vi "5492_WPI_RobotDriveArcadeDrive_Standard(NoSaturation).vi"(0 "RobotDriveDevRef":T1={"DevStatus"={"status"=FALSE, "code"=0, "source"=""}, "Motors[]"=[], "Square Inputs"=FALSE, "Max Output"=1.0}, 5 "X axis value":dbl, 7 "Orientation Toggle":bool, 9 "Y axis value":dbl, 11 "error in (no error)":errorcluster, 12 "Slow Toggle":bool) -> (4 "RobotDriveDevRef":T1={"DevStatus"={"status"=FALSE, "code"=0, "source"=""}, "Motors[]"=[], "Square Inputs"=FALSE, "Max Output"=1.0}, 6 "Motor Values":dbl[](array[numeric]), 15 "error out":errorcluster)   [LabVIEW 2017]
doc: "Uses a standard algorithm to configure the motors for arcade driving. This algorithm does not saturate over half of the range.\n\nThis software is licensed. Open the labview\\readme\\WPI Robotics Library Open Source License.txt file for more information."
uses:
  <vilib>/Rock Robotics/WPI/RobotDrive/WPI_RobotDriveDevRef.ctl
  <vilib>/Rock Robotics/WPI/MotorControl/WPI_MotorControlDeviceRef.ctl
  <vilib>/Rock Robotics/WPI/MotorControl/WPI_MotorControlType.ctl
  <vilib>/Rock Robotics/SystemInterfaces/DIO/FPGA_DIOPWMChannel.ctl
  <vilib>/Rock Robotics/WPI/PWM/WPI_PWMDeadband.ctl
  <vilib>/Rock Robotics/SystemInterfaces/DIO/FPGA_DIOChannel.ctl
  <vilib>/Rock Robotics/SystemInterfaces/NetworkCommunication/NetComm_UsageReport_ResourceType.ctl
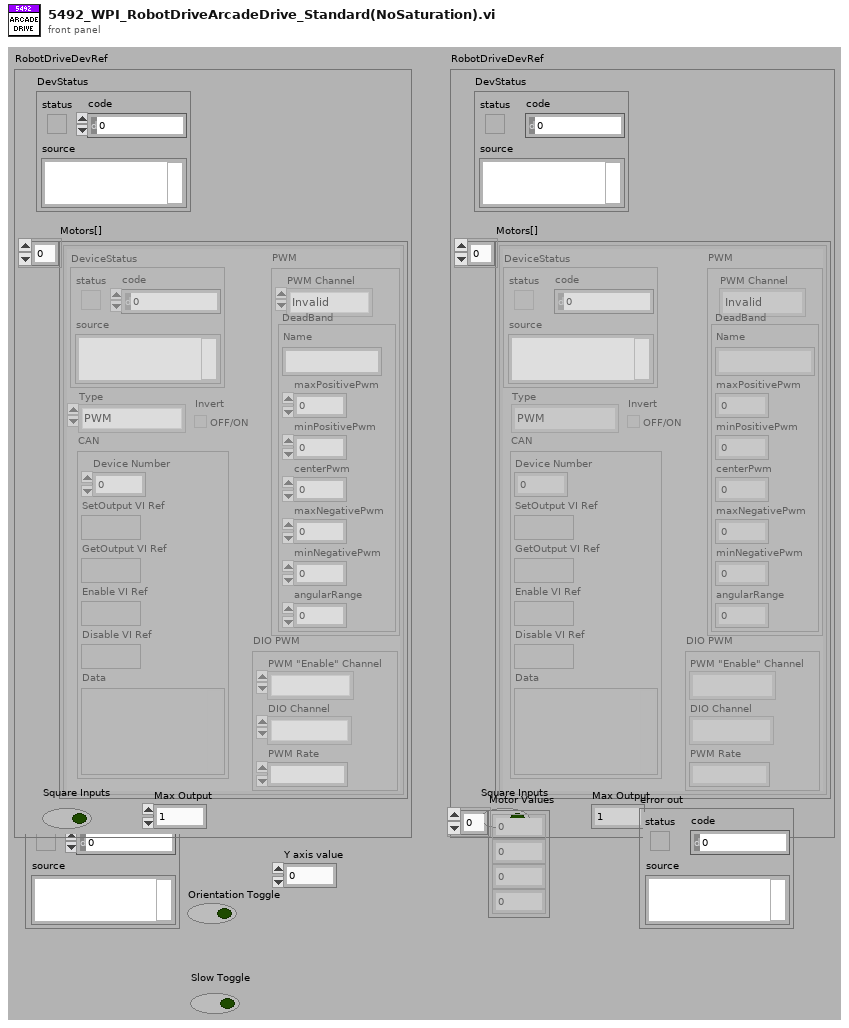
[diagram p1: front panel]
types:
  T1 = typedef "WPI_RobotDriveDevRef.ctl" = cluster{"DevStatus":errorcluster, "Motors[]":T2[], "Square Inputs":bool, "Max Output":dbl}
  T2 = typedef "WPI_MotorControlDeviceRef.ctl" = cluster{"DeviceStatus":errorcluster, "Type":T3, "PWM":cluster{"PWM Channel":T4, "DeadBand":T5}, "CAN":cluster{"Device Number":u8, "SetOutput VI Ref":variant, "GetOutput VI Ref":variant, "Enable VI Ref":variant, "Disable VI Ref":variant, "Data":variant}, "Invert":bool, "DIO PWM":cluster{"PWM \"Enable\" Channel":T4, "DIOChannel":T6, "PWM Rate":dbl}}
  T3 = typedef "WPI_MotorControlType.ctl" = enum16{"PWM", "CAN", "DIO PWM"}
  T4 = typedef "FPGA_DIOPWMChannel.ctl" = enum8{"PWM 0", "PWM 1", "PWM 2", "PWM 3", "PWM 4", "PWM 5", "PWM 6", "PWM 7", "PWM 8", "PWM 9", "PWM MXP 0", "PWM MXP 1", "PWM MXP 2", "PWM MXP 3", "PWM MXP 4", "PWM MXP 5", "PWM MXP 6", "PWM MXP 7", "PWM MXP 8", "PWM MXP 9", "Invalid"}
  T5 = typedef "WPI_PWMDeadband.ctl" = cluster{"Name":string, "maxPositivePwm":i32, "minPositivePwm":i32, "centerPwm":i32, "maxNegativePwm":i32, "minNegativePwm":i32, "angularRange":u16}
  T6 = typedef "FPGA_DIOChannel.ctl" = enum8{"DIO 0", "DIO 1", "DIO 2", "DIO 3", "DIO 4", "DIO 5", "DIO 6", "DIO 7", "DIO 8", "DIO 9", "DIO MXP 0", "DIO MXP 1", "DIO MXP 2", "DIO MXP 3", "DIO MXP 4", "DIO MXP 5", "DIO MXP 6", "DIO MXP 7", "DIO MXP 8", "DIO MXP 9", "DIO MXP 10", "DIO MXP 11", "DIO MXP 12", "DIO MXP 13", "DIO MXP 14", "DIO MXP 15", "SPI Port CS1", "SPI Port CS2", "SPI Port CS3", "SPI Port MISO", "SPI Port MOSI", "Invalid"}
  T7 = typedef "NetComm_UsageReport_ResourceType.ctl" = enum8{"Controller", "Module", "Language", "CANPlugin", "Accelerometer", "ADXL345", "AnalogChannel", "AnalogTrigger", "AnalogTriggerOutput", "CANJaguar", "Compressor", "Counter", "Dashboard", "DigitalInput", "DigitalOutput", "DriverStationCIO", "DriverStationEIO", "DriverStationLCD", "Encoder", "GearTooth", "Gyro", "I2C", "Framework", "Jaguar", "Joystick", "Kinect", "KinectStick", "PIDController", "Preferences", "PWM", "Relay", "RobotDrive", "SerialPort", "Servo", "Solenoid", "SPI", "Task", "Ultrasonic", "Victor", "Button", "Command", "AxisCamera", "PCVideoServer", "SmartDashboard", "Talon", "HiTechnicColorSensor", "HiTechnicAccel", "HiTechnicCompass", "SRF08", "AnalogOutput", "Victor SP", "Talon SRX", "CAN Talon SRX", "ADXL362 Accel", "ADXRS450 Gyro", "Rev SPARK", "Mindsensors SD540", "Digital Filter", "ADIS16448", "PDP", "PCM", "PigeonIMU", "Nidec Brushless", "CTRE CANifier", "CTRE Future 0", "CTRE Future 1", "CTRE Future 2", "CTRE Future 3", "CTRE Future 4", "CTRE Future 5", "CTRE Future 6"}
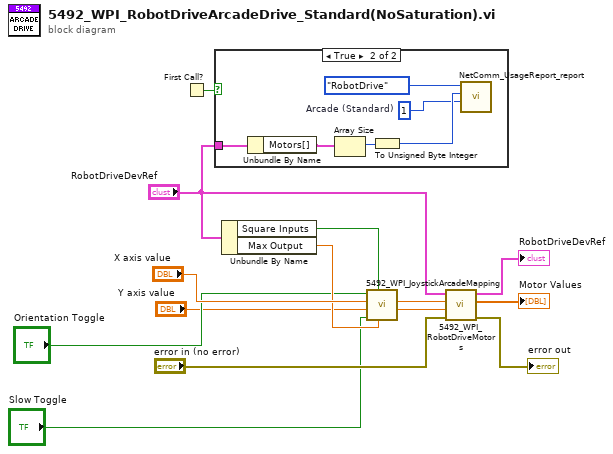
[diagram p0: block diagram]
diagram:
  n1 = First Call?() -> (First Call?: T/F=w11:bool)
  n2 = case shown="True" w11 {
    tunnel: "RobotDriveDevRef" -> [_ w16]
    frame False {
    }
    frame True {
      w18 = u8 1  # Arcade (Standard)
      n3 = Unbundle By Name(w16) -> ("Motors[]"=w15:T2[])
      n4 = Array Size(array=w15) -> (size(s)=w17:i32)
      n5 = To Unsigned Byte Integer(number=w17) -> (unsigned 8bit integer=w19:u8)
      n6 = call <vilib>:"NetComm_UsageReport_report.vi"("Context"=w18, "Instance Number"=w19, "Resource Type"=NetComm_UsageReport_ResourceType."RobotDrive") -> ()  [unwired: 9 in]
    }
  }
  n7 = Unbundle By Name("RobotDriveDevRef") -> ("Square Inputs"=w7:bool, "Max Output"=w5:dbl)
  n8 = call "5492_WPI_JoystickArcadeMapping.vi"("Max Output"=w5, "Square Inputs"=w7, "Slow Toggle"="Slow Toggle", "Y axis value"="Y axis value", "X axis value"="X axis value", "Orientation Toggle"="Orientation Toggle") -> ("Right Motor Value"=w8:dbl, "Left Motor Value"=w9:dbl)  [unwired: 4 in]
  n9 = call "5492_WPI_RobotDriveMotors.vi"("error in (no error)"="error in (no error)", "RightSpeed"=w8, "LeftSpeed"=w9, "RobotDriveDevRef"="RobotDriveDevRef") -> ("error out"=→"error out":errorcluster, "Motor Values"=→"Motor Values":dbl[], "RobotDriveDevRef"=→"RobotDriveDevRef":T1)  [unwired: 5 out]
